vi "LAB7.vi"() -> ()   [LabVIEW 2011]
uses:
  <userlib>/KNR LabVIEW Toolkit/Type Definitions/Port Number (for US).ctl
  <userlib>/KNR LabVIEW Toolkit/Type Definitions/Port Number (for DC).ctl
  <userlib>/KNR LabVIEW Toolkit/General/KNR Open (Direct Mode).vi
  <userlib>/KNR LabVIEW Toolkit/DC Motor Control/DC Motor Library.lvlib
  <userlib>/KNR LabVIEW Toolkit/Ultrasonic Control/Ultrasonic Library.lvlib
panel:
  out "Image Out":T1(plugin-control)
  out "Image Out 2":T1(plugin-control)
  out "Area size":dbl
  out "X":dbl
  in  "Port Number":T2 items=["US1-US4"=0, "US5-US8"=2]
  out "Ultrasonic output":T3
  out "right dis":dbl
  out "right Velocity (cts/sec) 2":dbl
  out "left Velocity (cts/sec)":dbl
  in  "Reverse Encoder 2":bool
  in  "Reset Encoder 2":bool
  in  "Reverse Encoder":bool
  in  "Reset Encoder":bool
  in  "Enable Motor":bool
  out "error out":errorcluster
  in  "stop":bool
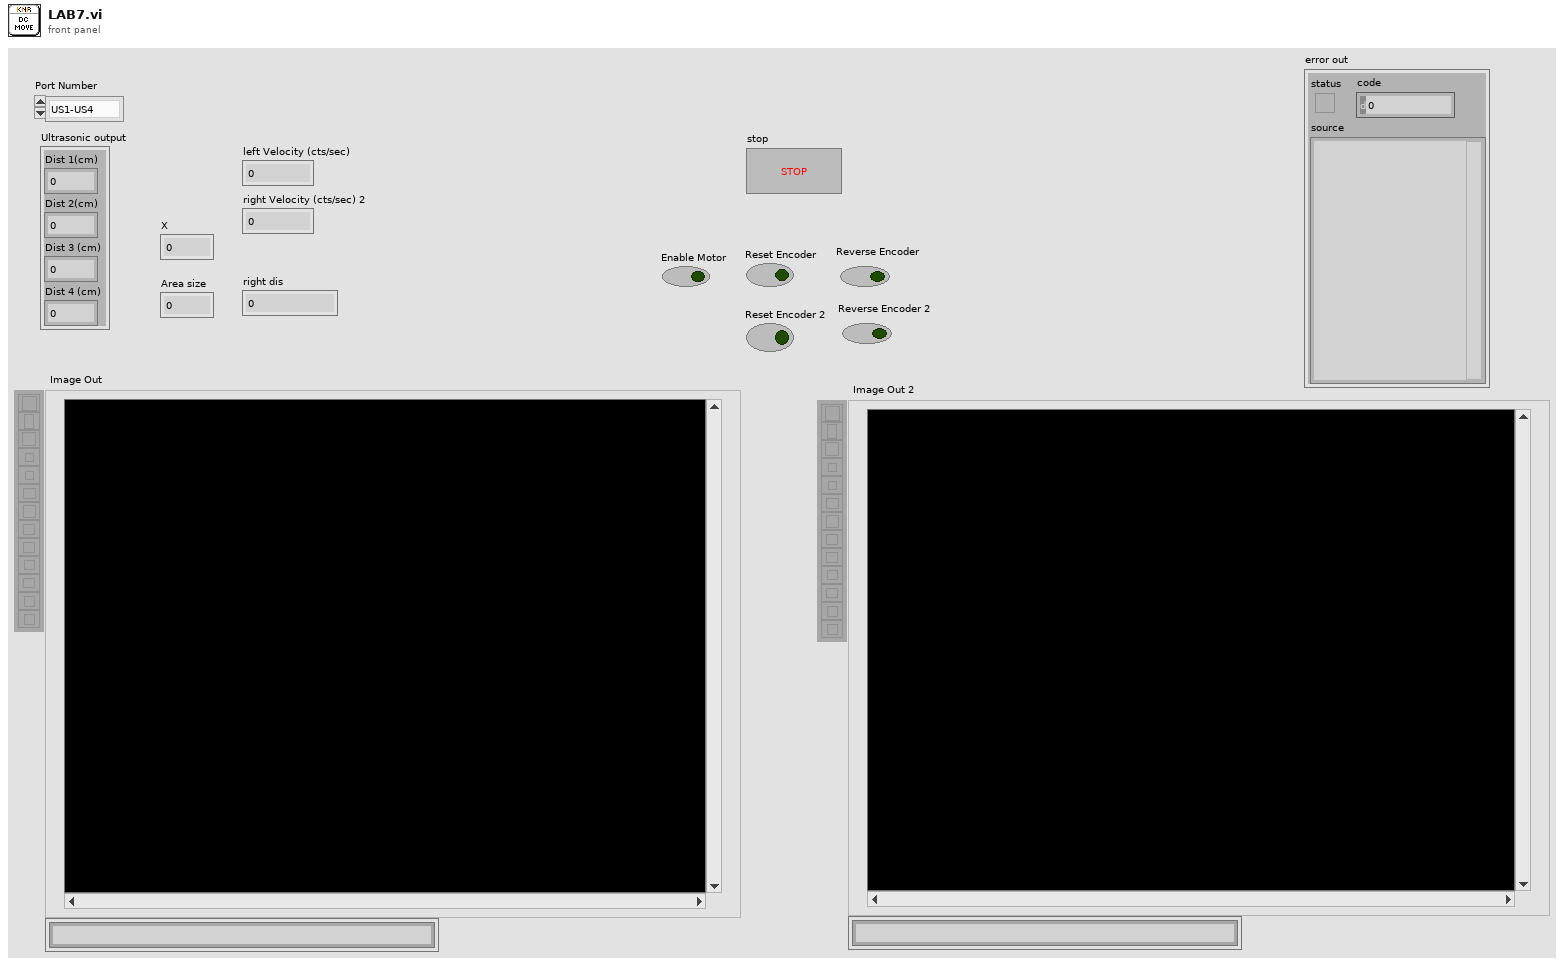
[diagram p1: front panel]
types:
  T1 = typedef "IMAQ Image.ctl" = refnum<image>
  T2 = typedef "Port Number (for US).ctl" = u16
  T3 = cluster{"Dist 1(cm)":dbl, "Dist 2(cm)":dbl, "Dist 3 (cm)":dbl, "Dist 4 (cm)":dbl}
  T4 = typedef "KNR Reference.ctl" = cluster{"FPGA Session":refnum<class "FPGA Interface Base.lvclass">, "Port Types":T5[]}
  T5 = typedef "Port Type (API).ctl" = enum8{"Unassigned", "DIO", "DC Motor", "RC Motor", "Ultrasonic", "Analog Input"}
  T6 = typedef "Port Number (for DC).ctl" = u16
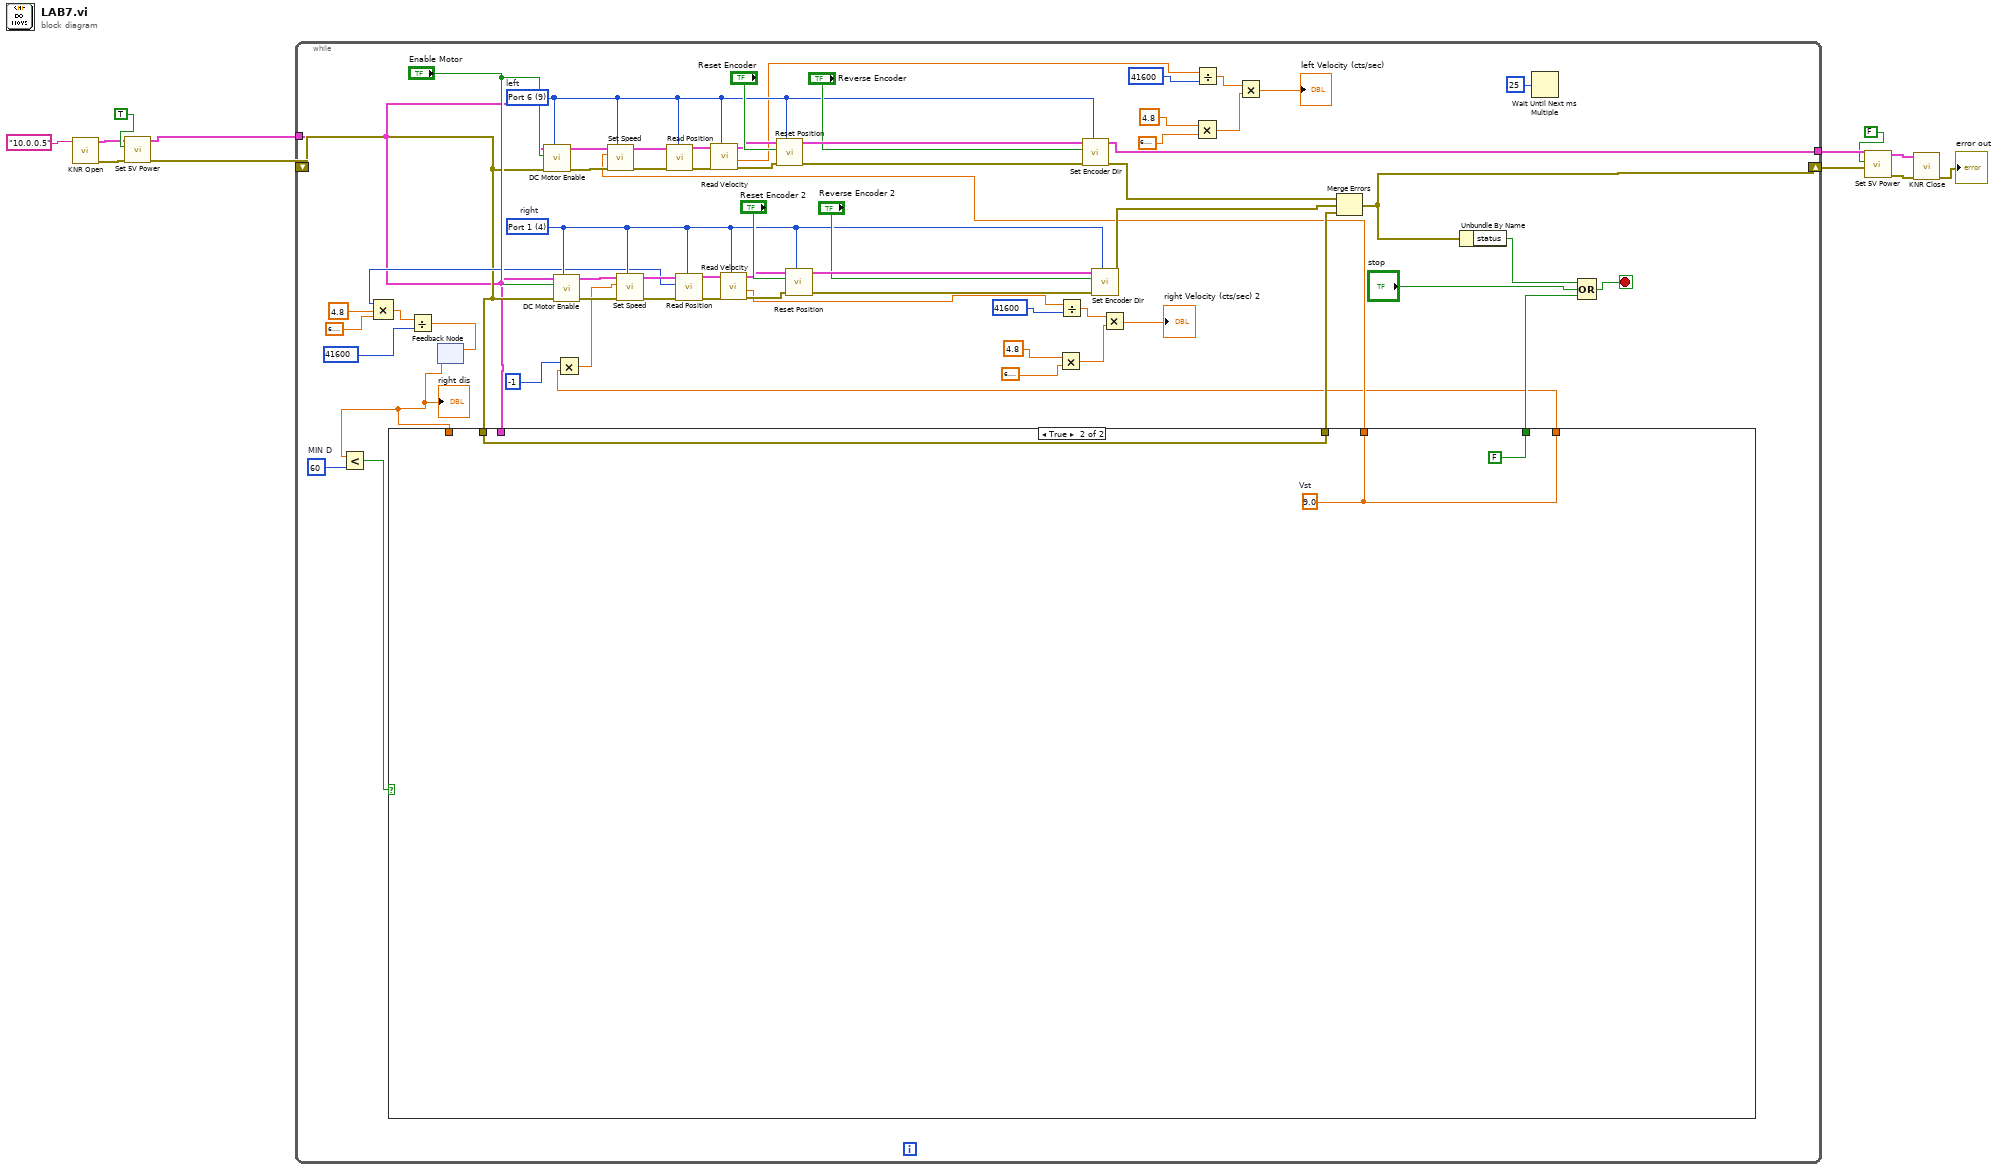
[diagram p0: block diagram]
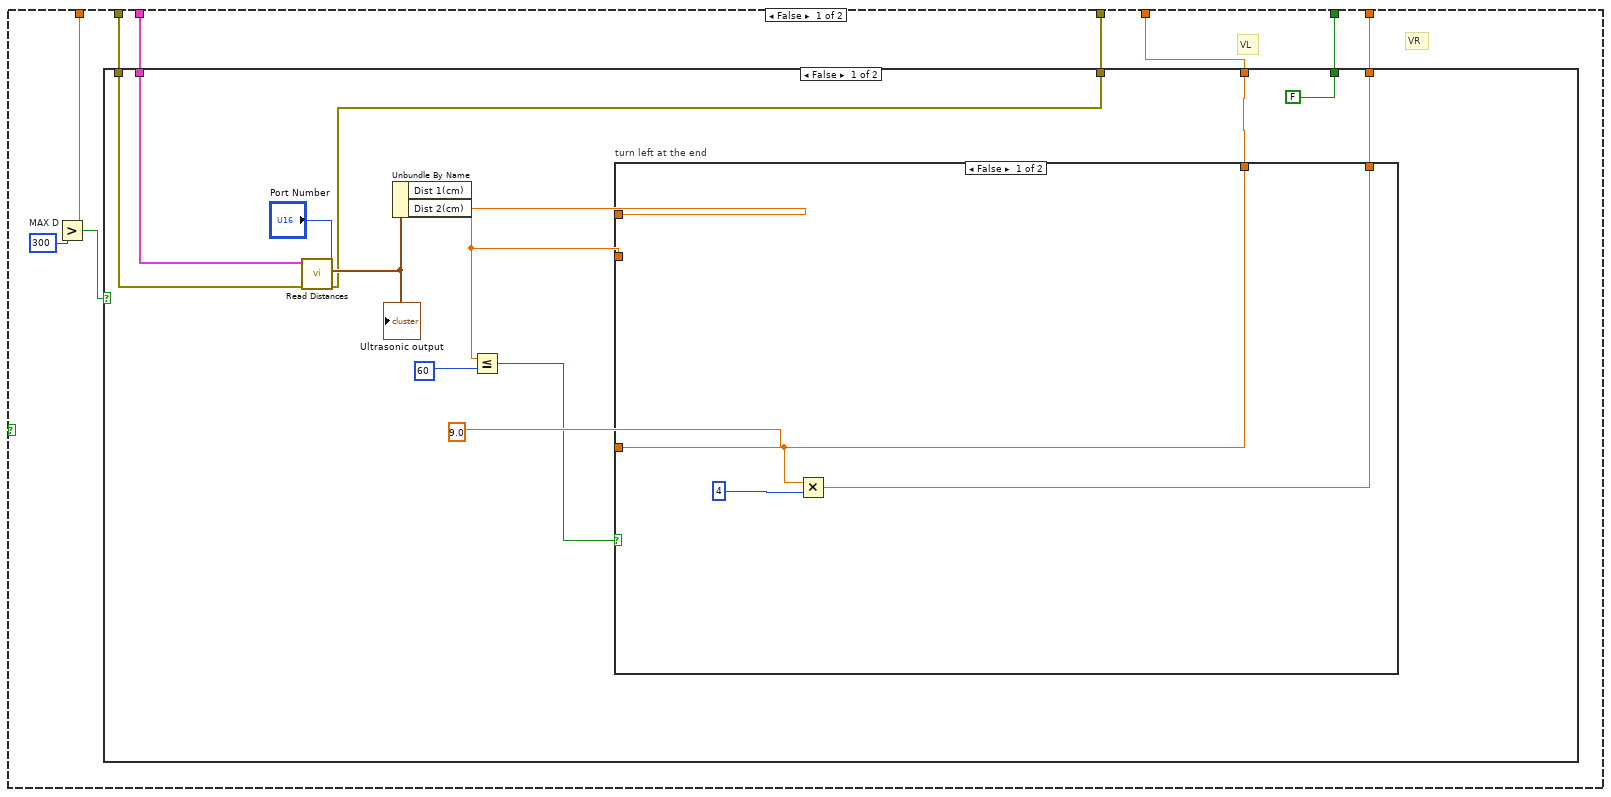
[diagram p2: hidden frame]
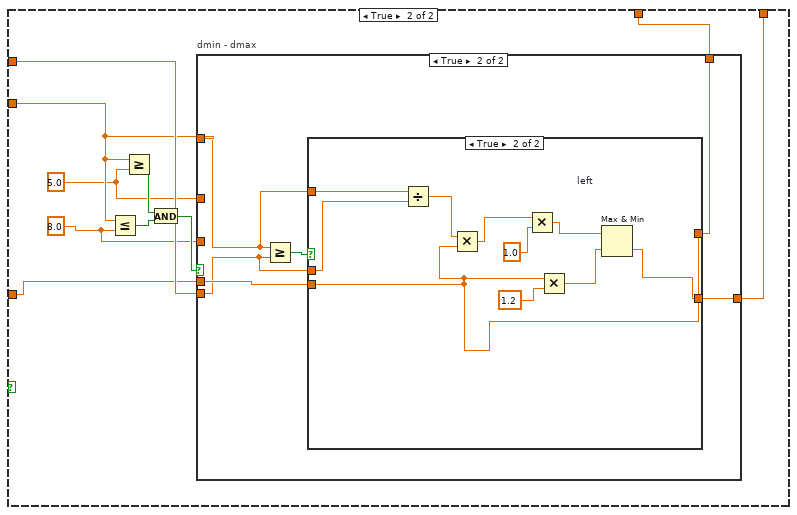
[diagram p3: hidden frame]
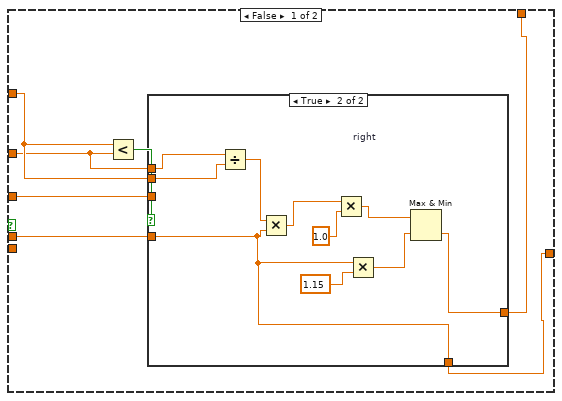
[diagram p4: hidden frame]
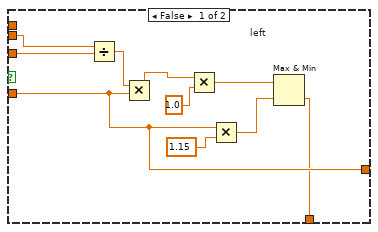
[diagram p5: hidden frame]
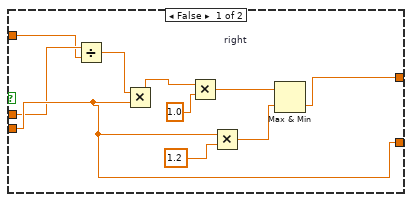
[diagram p6: hidden frame]
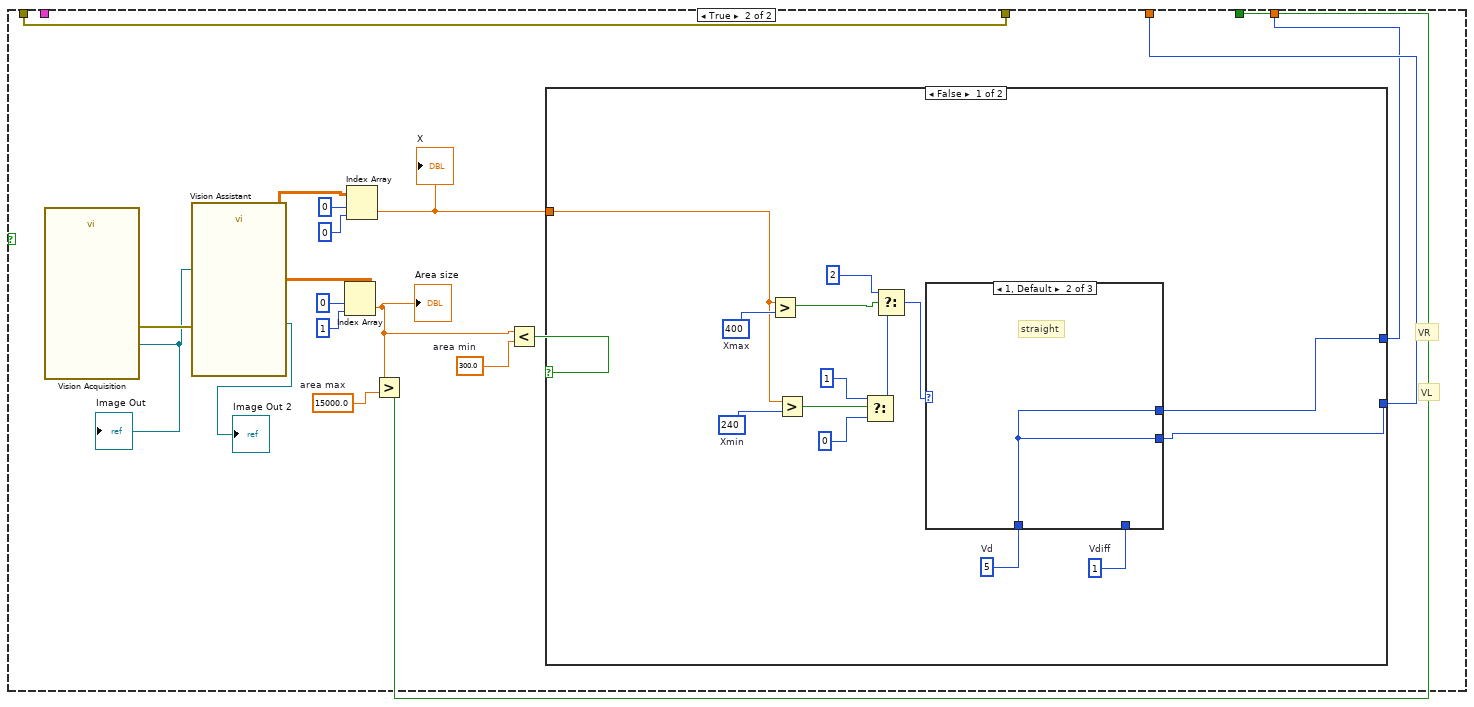
[diagram p7: hidden frame]
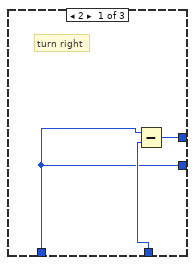
[diagram p8: hidden frame]
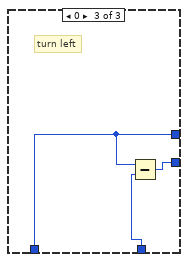
[diagram p9: hidden frame]
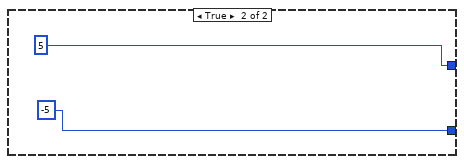
[diagram p10: hidden frame]
diagram:
  n1 = call-poly <userlib>:"KNR Open.vi"("IP Address (Default: 10.0.0.5)"="10.0.0.5") -> ("error out"=w1:errorcluster, "KNR Out"=w2:T4)  [unwired: 9 in]
  n2 = call <userlib>:"Set 5V Power.vi"("error in (no error)"=w1, "5V Power"=TRUE, "KNR In"=w2) -> ("error out"=w4:errorcluster, "KNR Out"=w5:T4)  [unwired: 7 in]
  n3 = while {
    shift-right: [w48] -> w9
    shift-left: w4 -> [w19]
    tunnel: [w52] -> w8
    tunnel: w5 -> [w17]
    stop <- w46 stop-if-true
    w21 = 60  # MIN D
    w60 = T6 4 items=["Port 1"=4, "Port 2"=5, "Port 3"=6, "Port 4"=7, "Port 5"=8, "Port 6"=9, "Port 7"=10]  # right
    w72 = T6 9 items=["Port 1"=4, "Port 2"=5, "Port 3"=6, "Port 4"=7, "Port 5"=8, "Port 6"=9, "Port 7"=10]  # left
    n4 = feedback #1() -> (w13:dbl)  [unwired: 1 in]
    "right dis" <- w13
    n5 = Less?(x=w13, y=w21) -> (x < y?=w20:bool)
    n6 = case shown="True" w20 {
      tunnel: w13 -> [w86 _]
      tunnel: w19 -> [w85 w207]
      tunnel: [w84 w207] -> w18
      tunnel: w17 -> [w83 _]
      tunnel: [w82 FALSE ("5V Power")] -> w16
      tunnel: [w81 w208] -> w15
      tunnel: [w80 w208] -> w14
      frame False {
        w87 = 300  # MAX D
        # "VL"
        # "VR"
        n7 = Greater?(x=w86, y=w87) -> (0:w79:bool)
        n8 = case shown="False" w79 {
          tunnel: [w93 w170] -> w81
          tunnel: [w92 w169] -> w80
          tunnel: [FALSE ("5V Power") w173] -> w82
          tunnel: w85 -> [w90 w168]
          tunnel: [w89 w168] -> w84
          tunnel: w83 -> [w88 _]
          frame False {
            n9 = call <userlib>:"Read Distances.vi"("Port Number"="Port Number", "error in (no error)"=w90, "KNR In"=w88) -> ("error out"=w89:errorcluster, "Ultrasonic output"=w99:T3)  [unwired: 6 in, 1 out]
            "Ultrasonic output" <- w99
            n10 = Unbundle By Name(w99) -> ("Dist 1(cm)"=w94:dbl, "Dist 2(cm)"=w95:dbl)
            n11 = Less Or Equal?(x=w94, y=60) -> (x <= y?=w97:bool)
            n12 = case "turn left at the end" shown="False" w97 {
              tunnel: w94 -> [_ w110]
              tunnel: [w103 w111] -> w93
              tunnel: 9.0 ("V") -> [w103 w112]
              tunnel: w95 -> [_ w113]
              tunnel: [w101 w104] -> w92
              frame False {
                n13 = Multiply(x=w103, y=4) -> (x*y=w101:dbl)
              }
              frame True {
                w105 = 8.0 ("D max")
                w106 = 5.0 ("D max")
                n14 = Less Or Equal?(x=w110, y=w105) -> (x <= y?=w108:bool)
                n15 = Greater Or Equal?(x=w110, y=w106) -> (x >= y?=w109:bool)
                n16 = And(x=w109, y=w108) -> (x .and. y?=w107:bool)
                n17 = case "dmin - dmax" shown="True" w107 {
                  tunnel: w110 -> [w119 w145]
                  tunnel: w113 -> [_ w142]
                  tunnel: w106 -> [w116 _]
                  tunnel: w112 -> [w118 w144]
                  tunnel: [w115 w143] -> w111
                  tunnel: w105 -> [w117 _]
                  tunnel: [w114 w141] -> w104
                  frame False {
                    n18 = Less?(x=w119, y=w116) -> (x < y?=w120:bool)
                    n19 = case shown="True" w120 {
                      tunnel: w119 -> [w123 w131]
                      tunnel: w118 -> [w125 w133]
                      tunnel: w117 -> [w122 _]
                      tunnel: w116 -> [_ w132]
                      tunnel: [w125 w134] -> w115
                      tunnel: [w121 w133] -> w114
                      frame False {
                        n20 = Divide(x=w123, y=w122) -> (x/y=w129:dbl)
                        n21 = Multiply(x=w129, y=w125) -> (x*y=w128:dbl)
                        n22 = Multiply(x=w128, y=1.0) -> (x*y=w126:dbl)
                        n23 = Multiply(x=w125, y=1.15) -> (x*y=w124:dbl)
                        n24 = Max & Min "left"(x=w126, y=w124) -> (min(x,y)=w121:dbl)  [unwired: 1 out]
                      }
                      frame True {
                        n25 = Divide(x=w132, y=w131) -> (x/y=w140:dbl)
                        n26 = Multiply(x=w140, y=w133) -> (x*y=w136:dbl)
                        n27 = Multiply(x=w136, y=1.0) -> (x*y=w135:dbl)
                        n28 = Multiply(x=w133, y=1.15) -> (x*y=w138:dbl)
                        n29 = Max & Min "right"(x=w135, y=w138) -> (min(x,y)=w134:dbl)  [unwired: 1 out]
                      }
                    }
                  }
                  frame True {
                    n30 = Greater Or Equal?(x=w145, y=w142) -> (x >= y?=w146:bool)
                    n31 = case shown="True" w146 {
                      tunnel: [w153 w159] -> w143
                      tunnel: [w149 w157] -> w141
                      tunnel: w145 -> [w147 w160]
                      tunnel: w144 -> [w149 w159]
                      tunnel: w142 -> [w148 w158]
                      frame False {
                        n32 = Divide(x=w148, y=w147) -> (x/y=w154:dbl)
                        n33 = Multiply(x=w154, y=w149) -> (x*y=w152:dbl)
                        n34 = Multiply(x=w152, y=1.0) -> (x*y=w150:dbl)
                        n35 = Multiply(x=w149, y=1.2) -> (x*y=w156:dbl)
                        n36 = Max & Min "right"(x=w150, y=w156) -> (min(x,y)=w153:dbl)  [unwired: 1 out]
                      }
                      frame True {
                        n37 = Divide(x=w160, y=w158) -> (x/y=w166:dbl)
                        n38 = Multiply(x=w166, y=w159) -> (x*y=w162:dbl)
                        n39 = Multiply(x=w162, y=1.0) -> (x*y=w161:dbl)
                        n40 = Multiply(x=w159, y=1.2) -> (x*y=w164:dbl)
                        n41 = Max & Min "left"(x=w161, y=w164) -> (min(x,y)=w157:dbl)  [unwired: 1 out]
                      }
                    }
                  }
                }
              }
            }
          }
          frame True {
            w179 = 300.0  # area min
            w180 = 15000.0  # area max
            # "VL"
            # "VR"
            n42 = call "Vision Acquisition"() -> ("Image Out"=w182:T1, "error out"=w183:errorcluster)  [unwired: 25 in, 1 out]
            "Image Out" <- w182
            n43 = call "Vision Assistant"("Image In"=w182, "error in"=w183) -> ("Image Out"=→"Image Out 2":T1, "Particle Measurements (Pixels) (Particle Analysis 1)"=w175:dbl[][])  [unwired: 23 in, 1 out]
            n44 = Index Array(array=w175, index (row)=0 ("index"), index (col)=1 ("index")) -> (element=w174:dbl)
            "Area size" <- w174
            n45 = Index Array(array=w175, index (row)=0 ("index"), index (col)=0 ("index")) -> (element=w171:dbl)
            "X" <- w171
            n46 = Greater?(x=w174, y=w180) -> (0:w173:bool)
            n47 = Less?(x=w174, y=w179) -> (x < y?=w172:bool)
            n48 = case shown="False" w172 {
              tunnel: [w185 5] -> w169
              tunnel: [w184 -5] -> w170
              tunnel: w171 -> [w186 _]
              frame False {
                w188 = 1  # Vdiff
                w189 = 5  # Vd
                w197 = 240  # Xmin
                w196 = 400  # Xmax
                n49 = Greater?(x=w186, y=w196) -> (0:w190:bool)
                n50 = Greater?(x=w186, y=w197) -> (0:w193:bool)
                n51 = Select(t=1, s=w193, f=0) -> (s? t:f=w191:i32)
                n52 = Select(t=2, s=w190, f=w191) -> (s? t:f=w187:i32)
                n53 = case shown="1, Default" w187 {
                  tunnel: w189 -> [w199 w201 w204]
                  tunnel: w188 -> [w200 _ w203]
                  tunnel: [w199 w201 w202] -> w184
                  tunnel: [w198 w201 w204] -> w185
                  frame 2 {
                    # "turn right"
                    n54 = Subtract(x=w199, y=w200) -> (x-y=w198:i32)
                  }
                  frame 1, Default {
                    # "straight"
                  }
                  frame 0 {
                    # "turn left"
                    n55 = Subtract(x=w204, y=w203) -> (x-y=w202:i32)
                  }
                }
              }
              frame True {
              }
            }
          }
        }
      }
      frame True {
        w208 = 9.0  # Vst
      }
    }
    n56 = call <userlib>:"DC Motor Enable.vi"("Port Number"=w72, "error in (no error)"=w19, "Enable Motor"="Enable Motor", "KNR In"=w17) -> ("error out"=w73:errorcluster, "KNR Out"=w74:T4)  [unwired: 6 in]
    n57 = call <userlib>:"DC Motor Enable.vi"("Port Number"=w60, "error in (no error)"=w19, "Enable Motor"="Enable Motor", "KNR In"=w17) -> ("error out"=w61:errorcluster, "KNR Out"=w62:T4)  [unwired: 6 in]
    n58 = Multiply(x=-1, y=w14) -> (x*y=w38:dbl)
    n59 = call <userlib>:"Set Speed.vi"("Port Number"=w72, "error in (no error)"=w73, "Speed (+-100%)"=w15, "KNR In"=w74) -> ("error out"=w70:errorcluster, "KNR Out"=w71:T4)  [unwired: 6 in]
    n60 = call <userlib>:"Set Speed.vi"("Port Number"=w60, "error in (no error)"=w61, "Speed (+-100%)"=w38, "KNR In"=w62) -> ("error out"=w58:errorcluster, "KNR Out"=w59:T4)  [unwired: 6 in]
    n61 = call <userlib>:"Read Position.vi"("Port Number"=w72, "error in (no error)"=w70, "KNR In"=w71) -> ("error out"=w68:errorcluster, "KNR Out"=w69:T4)  [unwired: 6 in, 1 out]
    n62 = call <userlib>:"Read Position.vi"("Port Number"=w60, "error in (no error)"=w58, "KNR In"=w59) -> ("error out"=w56:errorcluster, "Position"=w22:i32, "KNR Out"=w57:T4)  [unwired: 6 in]
    n63 = Compound Arithmetic op=MULTIPLY(w22, 4.8, 6.283185307179586) -> (w42:dbl)
    n64 = Divide(x=w42, y=41600) -> (x/y=w41:dbl)
    n65 = feedback-in #1(w41) -> ()
    n66 = call <userlib>:"Read Velocity.vi"("Port Number"=w72, "error in (no error)"=w68, "KNR In"=w69) -> ("error out"=w66:errorcluster, "Velocity (cts/sec)"=w24:dbl, "KNR Out"=w67:T4)  [unwired: 6 in]
    n67 = call <userlib>:"Read Velocity.vi"("Port Number"=w60, "error in (no error)"=w56, "KNR In"=w57) -> ("error out"=w54:errorcluster, "Velocity (cts/sec)"=w23:dbl, "KNR Out"=w55:T4)  [unwired: 6 in]
    n68 = call <userlib>:"Reset Position.vi"("Port Number"=w72, "error in (no error)"=w66, "Reset"="Reset Encoder", "KNR In"=w67) -> ("error out"=w77:errorcluster, "KNR Out"=w78:T4)  [unwired: 6 in]
    n69 = call <userlib>:"Reset Position.vi"("Port Number"=w60, "error in (no error)"=w54, "Reset"="Reset Encoder 2", "KNR In"=w55) -> ("error out"=w45:errorcluster, "KNR Out"=w65:T4)  [unwired: 6 in]
    n70 = Multiply(x=4.8, y=6.283185307179586) -> (x*y=w28:dbl)
    n71 = Divide(x=w23, y=41600) -> (x/y=w30:dbl)
    n72 = call <userlib>:"Set Encoder Dir.vi"("Port Number"=w72, "error in (no error)"=w77, "Reverse?"="Reverse Encoder", "KNR In"=w78) -> ("error out"=w51:errorcluster, "KNR Out"=w52:T4)  [unwired: 6 in]
    n73 = call <userlib>:"Set Encoder Dir.vi"("Port Number"=w60, "error in (no error)"=w45, "Reverse?"="Reverse Encoder 2", "KNR In"=w65) -> ("error out"=w50:errorcluster)  [unwired: 6 in, 1 out]
    n74 = Multiply(x=w30, y=w28) -> (x*y=→"right Velocity (cts/sec) 2":dbl)
    n75 = Multiply(x=4.8, y=6.283185307179586) -> (x*y=w33:dbl)
    n76 = Divide(x=w24, y=41600) -> (x/y=w36:dbl)
    n77 = Multiply(x=w36, y=w33) -> (x*y=→"left Velocity (cts/sec)":dbl)
    n78 = Merge Errors(w51, w50, w18) -> (w48:errorcluster)
    n79 = Unbundle By Name(w48) -> ("status"=w47:bool)
    n80 = Wait Until Next ms Multiple(millisecond multiple=u32 25) -> ()  [unwired: 1 out]
    n81 = Compound Arithmetic op=OR(w47, "stop", w16) -> (w46:bool)
  }
  n82 = call <userlib>:"Set 5V Power.vi"("error in (no error)"=w9, "5V Power"=FALSE, "KNR In"=w8) -> ("error out"=w11:errorcluster, "KNR Out"=w12:T4)  [unwired: 7 in]
  n83 = call <userlib>:"KNR Close.vi"("error in (no error)"=w11, "KNR In"=w12) -> ("error out"=→"error out":errorcluster)  [unwired: 9 in]
